vi "aoc-2025-d06-1.vi"() -> ()   [LabVIEW 2020]
panel:
  out "sum":i64
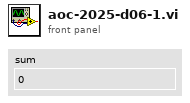
[diagram p1: front panel]
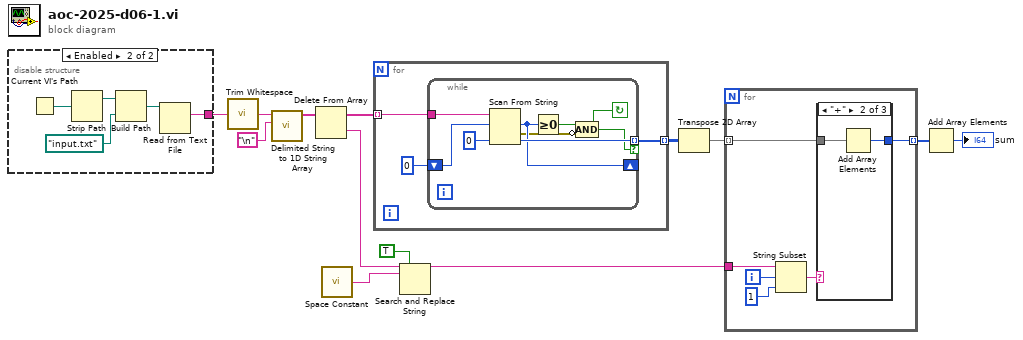
[diagram p0: block diagram]
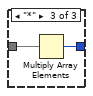
[diagram p3: hidden frame]
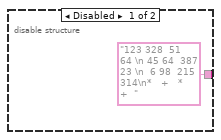
[diagram p4: hidden frame]
diagram:
  n1 = disable-structure shown="Enabled" {
    disable-tunnel: ["123 328  51 64 \n 45 64  387 23 \n  6 98  215 314\n*   +   *   +  " w15] -> w13
    frame Disabled {
    }
    frame Enabled {
      n2 = Current VI's Path() -> (path=w17:path)
      n3 = Strip Path(path=w17) -> (stripped path=w18:path)  [unwired: 1 out]
      n4 = Build Path(base path=w18, name or relative path=path "input.txt") -> (appended path=w19:path)
      n5 = Read from Text File(file (use dialog)=w19) -> (text=w15:string)  [unwired: 3 in, 3 out]
    }
  }
  n6 = call <vilib>:"Trim Whitespace.vi"("string"=w13) -> ("trimmed string"=w12:string)  [unwired: 1 in]
  n7 = call <vilib>:"Delimited String to 1D String Array.vi"("delimiter"="\n", "delimited string"=w12) -> ("string array"=w7:string[])  [unwired: 9 in]
  n8 = Delete From Array(array=w7) -> (deleted portion=w11:string, array with subset deleted=w8:string[])  [unwired: 2 in]
  n9 = call <vilib>:"Space Constant.vi"() -> ("String"=w10:string)
  n10 = for {
    tunnel: w8 -> [w20] mode=indexing
    tunnel: [w21] -> w1 mode=indexing
    n11 = while {
      tunnel: w20 -> [w30]
      tunnel: [w27] -> w21 mode=indexing if=w23
      shift-right: [w26] -> _
      shift-left: u32 0 -> [w25]
      stop <- w23 continue-if-true
      n12 = Scan From String(input string=w30, initial scan location=w25, default 1=i64 0) -> (offset past scan=w26:u32, error out=w24:errorcluster, output 1=w27:i64)  [unwired: 2 in, 1 out]
      n13 = Greater Or Equal To 0?(x=w26) -> (x >= 0?=w28:bool)
      n14 = Compound Arithmetic op=AND(w28, invert w24) -> (w23:bool)
    }
  }
  n15 = Search and Replace String(replace all?=TRUE ("replace all? (F)"), input string=w11, search string=w10) -> (result string=w4:string)  [unwired: 5 in, 3 out]
  n16 = Transpose 2D Array(2D array=w1) -> (transposed array=w5:i64[][])
  n17 = for {
    tunnel: w5 -> [w32] mode=indexing
    tunnel: w4 -> [w36]
    tunnel: [w31] -> w3 mode=indexing
    i -> [w35]
    n18 = String Subset(string=w36, offset (0)=w35, length (rest)=1 ("length (rest)")) -> (substring=w33:string)
    n19 = case shown="\"+\"" w33 {
      tunnel: w32 -> [_ w38 w40]
      tunnel: [_ w37 w39] -> w31
      frame Default {
      }
      frame "+" {
        n20 = Add Array Elements(numeric array=w38) -> (sum=w37:i64)
      }
      frame "*" {
        n21 = Multiply Array Elements(1:w40) -> (0:w39:i64)
      }
    }
  }
  n22 = Add Array Elements(numeric array=w3) -> (sum=→"sum":i64)
